vi "SECADO_enterComms.vi"(8 "error in (no error)":errorcluster) -> (0 "error out":errorcluster, 2 "Cancelled?":bool, 3 "Comunicaciones":T1={"Eurotherm"="", "CDT"=FALSE, "Agilent"="ASRL6::INSTR", "AGL"=FALSE, "#Dec"=1} {"#Dec" items=["1"=1, "1"=10, "2"=100]})   [LabVIEW 2017]
doc: "Use this template to create a dialog box. This template polls the state of the buttons on the front panel and does not use events. Use the Dialog Using Events template (not available in Base package) to create a dialog box with event handling."
uses:
  Typedefs/SECADO_comms--Cluster.ctl
panel:
  in  "#dec":u16(ring)=1 items=["0", "1", "2"]
  in  "AGL":bool=TRUE
  in  "Agilent":refnum<visa-resource-name>="COM3"
  in  "CDT":bool=TRUE
  in  "Eurothem":refnum<visa-resource-name>="COM4"
  out "Si usado":bool=TRUE
  out "No usado":bool
  in  "Cancel":bool
  in  "OK":bool
  # "Configuración ...."
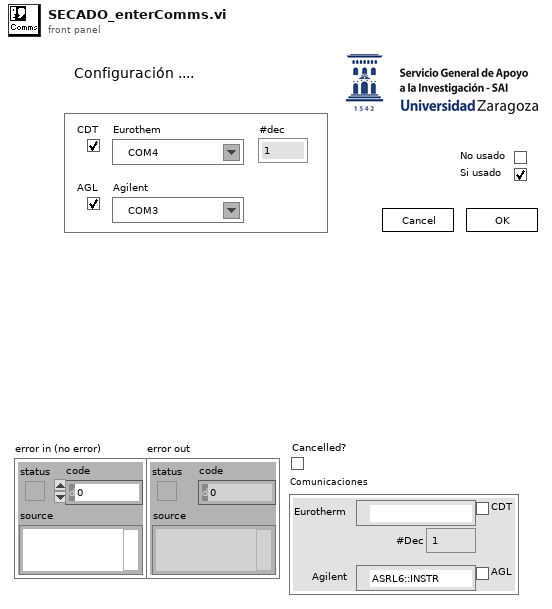
[diagram p1: front panel]
types:
  T1 = typedef "SECADO_comms--Cluster.ctl" = cluster{"Eurotherm":refnum<visa-resource-name>, "CDT":bool, "Agilent":refnum<visa-resource-name>, "AGL":bool, "#Dec":u16}
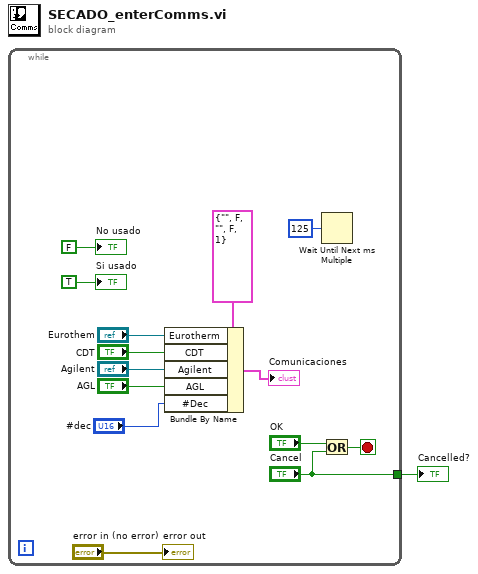
[diagram p0: block diagram]
diagram:
  n1 = while {
    tunnel: ["Cancel"] -> w1
    stop <- w14 stop-if-true
    n2 = Bundle By Name(cluster=T1 {"Eurotherm"="", "CDT"=FALSE, "Agilent"="", "AGL"=FALSE, "#Dec"=1} ("Comunicaciones"), "Eurotherm"="Eurothem", "CDT"="CDT", "Agilent"="Agilent", "AGL"="AGL", "#Dec"="#dec") -> (→"Comunicaciones":T1)
    n3 = Wait Until Next ms Multiple(millisecond multiple=u32 125) -> ()  [unwired: 1 out]
    n4 = Or(x="OK", y="Cancel") -> (x .or. y?=w14:bool)
    "error out" <- "error in (no error)"
    "No usado" <- FALSE ("No usado")
    "Si usado" <- TRUE ("Si usado")
  }
  "Cancelled?" <- w1
